vi "Driver Delete All.vi"(8 "error in (no error)":errorcluster, 11 "Connection Refnum":T1) -> (0 "error out":errorcluster, 3 "Connection Refnum":T1)   [LabVIEW 2011]
uses:
  SI.LIB/ODBC/SQL Controls/Connection Refnum.ctl
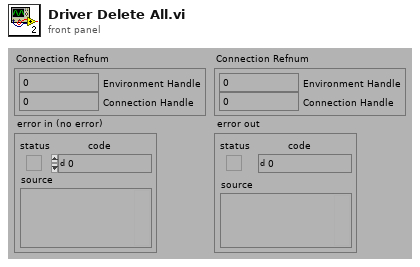
[diagram p1: front panel]
types:
  T1 = typedef "Connection Refnum.ctl" = cluster{"Environment Handle":i32, "Connection Handle":i32}
  T2 = typedef "Driver Record.ctl" = cluster{"ixDriver":i32, "sxDriverId":string, "sType":string, "sVersion":string}
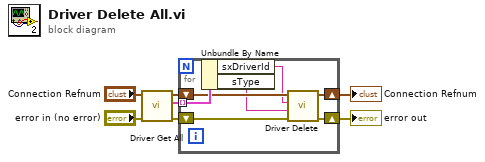
[diagram p0: block diagram]
diagram:
  n1 = call "Driver Get All.vi"("error in (no error)"="error in (no error)", "Connection Refnum"="Connection Refnum") -> ("error out"=w5:errorcluster, "Drivers"=w7:T2[], "Connection Refnum"=w6:T1)  [unwired: 2 in, 5 out]
  n2 = for {
    tunnel: w7 -> [w14] mode=indexing
    shift-right: [w11] -> w1
    shift-left: w5 -> [w12]
    shift-right: [w10] -> w2
    shift-left: w6 -> [w13]
    n3 = Unbundle By Name(w14) -> ("sxDriverId"=w9:string, "sType"=w8:string)
    n4 = call "Driver Delete.vi"("error in (no error)"=w12, "sType"=w8, "sxDriverId"=w9, "Connection Refnum"=w13) -> ("error out"=w11:errorcluster, "Connection Refnum"=w10:T1)  [unwired: 6 out]
  }
  "error out" <- w1
  "Connection Refnum" <- w2
